vi "Image Aqq IRC Test.vi"() -> (0 "Image":T1(plugin-control))   [LabVIEW 2015, in "Everything.lvlib"]
uses:
  Everything.lvlib
  <vilib>/userdefined/High Color/IMAQdx.ctl
panel:
  out "Image Name":string
  in  "Error In":errorcluster
  out "Error Out":errorcluster
  in  "Camera":T2
  in  "Stop Button":bool
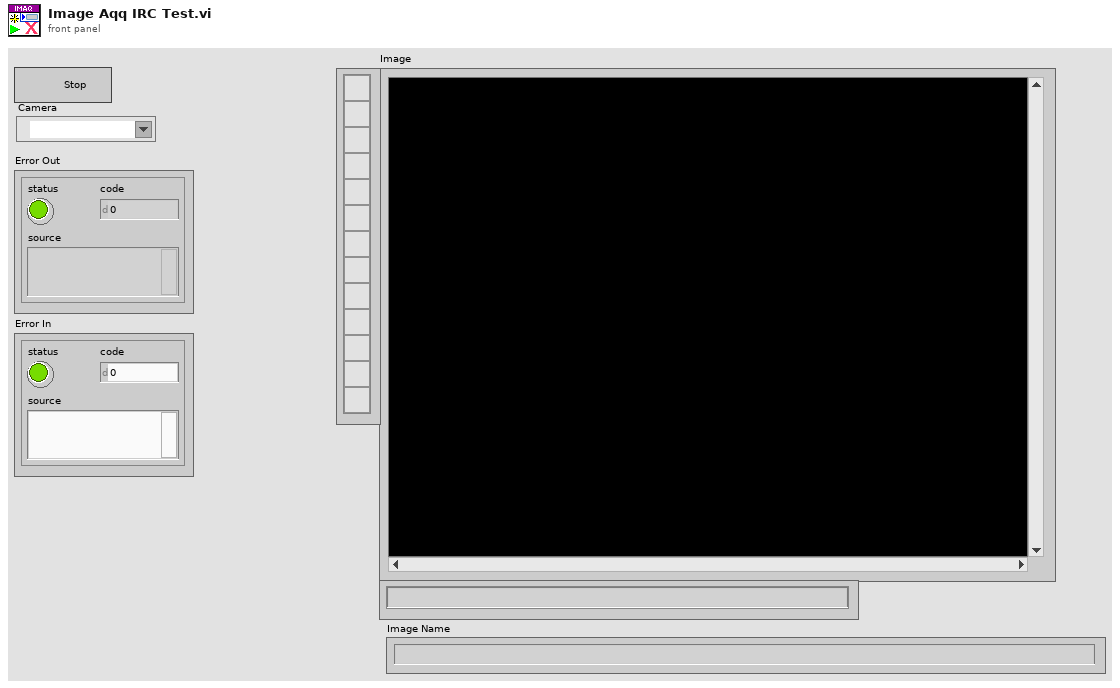
[diagram p1: front panel]
types:
  T1 = typedef "IMAQ Image.ctl" = refnum<image>
  T2 = typedef "IMAQdx.ctl" = refnum<k21>
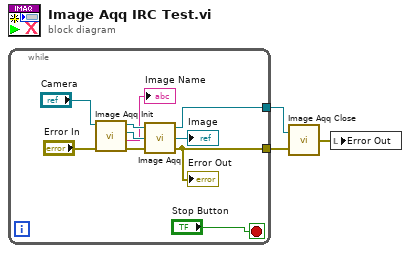
[diagram p0: block diagram]
diagram:
  n1 = while {
    tunnel: [w9] -> w3
    tunnel: [w8] -> w2
    stop <- "Stop Button" stop-if-true
    n2 = call "Image Aqq Init.vi"("Error In"="Error In", "Camera"="Camera") -> ("Error Out"=w13:errorcluster, "Image Name"=→"Image Name":string, "Img Out"=w12:T1, "Cam Out"=w11:T2)  [unwired: 6 in]
    n3 = call "Image Aqq.vi"("Error In"=w13, "Img In"=w12, "Session In"=w11) -> ("Error Out"=w8:errorcluster, "Image"=→"Image":T1, "Cam Out"=w9:T2)
    "Error Out" <- w8
  }
  n4 = call "Image Aqq Close.vi"("Error In"=w2, "Session In"=w3) -> ("Error Out"=w1:errorcluster)
  n5 = local write "Error Out"(w1) -> ()
